vi "Sqaure Number.vi"(8 "Error In":errorcluster, 11 "number in":i32) -> (0 "Error Out":errorcluster, 3 "number out":i32)   [LabVIEW 2014]
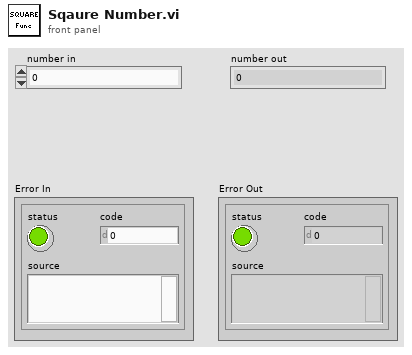
[diagram p1: front panel]
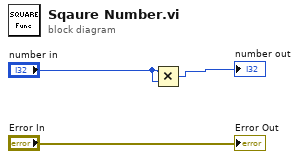
[diagram p0: block diagram]
diagram:
  n1 = Multiply(x="number in", y="number in") -> (x*y=→"number out":i32)
  "Error Out" <- "Error In"
